vi "test Add RAF Channel.vi"(8 "error in (no error)":errorcluster, 11 "TestCase in":refnum<class "Switch Scripting Unit Tests.lvclass">) -> (0 "error out":errorcluster, 3 "TestCase out":refnum<class "Switch Scripting Unit Tests.lvclass">)   [LabVIEW 2017, in "Switch Scripting.lvlib" / "Switch Scripting Unit Tests.lvclass"]
uses:
  Switch Scripting Unit Tests.lvclass
  Channel States.ctl
  Routing State.ctl
  Routing Channel/Connection.ctl
  Switch Scripting Unit Tests.lvclass/Switch Scripting Unit Tests.ctl
  <vilib>/addons/_JKI Toolkits/VI Tester/TestCase.llb/TestCase.lvclass
  Switch Scripting.lvlib
  C:/Program Files (x86)/National Instruments/LabVIEW 2017/vi.lib/addons/_JKI Toolkits/VI Tester/TestCase.llb/TestCase.lvclass
panel:
  in  "Save?":bool
  out "Output Filename":string
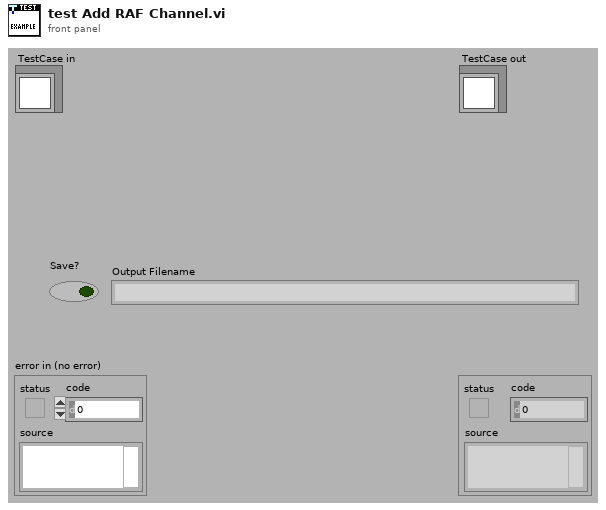
[diagram p1: front panel]
types:
  T1 = typedef "Switch Scripting.lvlib/Connection.ctl" = cluster{"source":string, "destination":string}
  T2 = typedef "Switch Scripting.lvlib/Channel States.ctl" = T3[]
  T3 = typedef "Switch Scripting.lvlib/Routing State.ctl" = cluster{"name":string, "description":string, "value":i32, "connection list":T1[]}
  T4 = typedef "Custom Device API.lvlib/Custom Device Item Ref.ctl" = u64
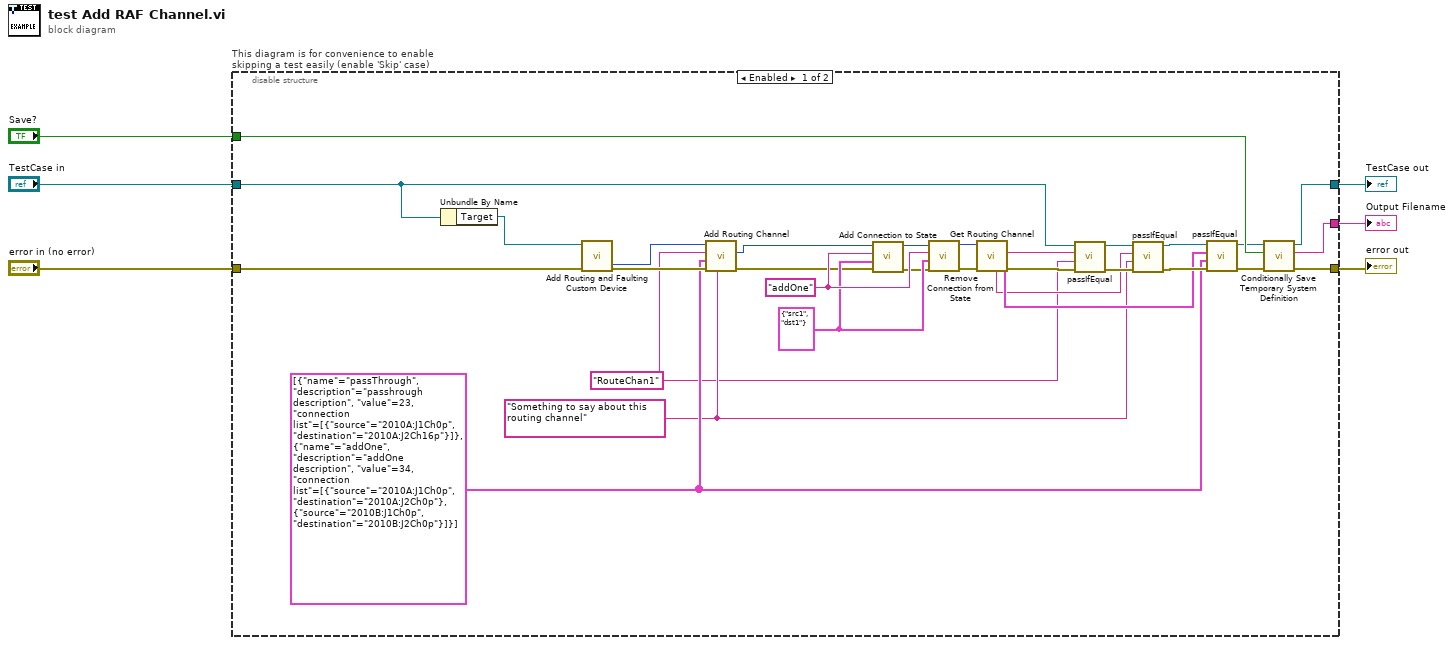
[diagram p0: block diagram]
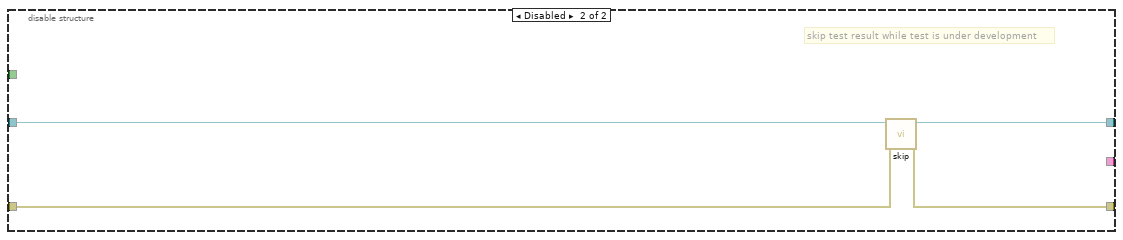
[diagram p2: hidden frame]
diagram:
  n1 = disable-structure "This diagram is for convenience to enable skipping a test easily (enable 'Skip' case)" shown="Enabled" {
    disable-tunnel: "TestCase in" -> [w16 w40]
    disable-tunnel: [w31 w38] -> w3
    disable-tunnel: [w35 w39] -> w5
    disable-tunnel: "error in (no error)" -> [w36 w37]
    disable-tunnel: [w34 _] -> w2
    disable-tunnel: "Save?" -> [w33 _]
    frame Enabled {
      w9 = "Something to say about this routing channel" ("Description")
      w25 = T1 {"source"="src1", "destination"="dst1"} ("connection")
      w26 = "addOne" ("state name")
      w11 = T2 [{"name"="passThrough", "description"="passhrough description", "value"=23, "connection list"=[{"source"="2010A:J1Ch0p", "destination"="2010A:J2Ch16p"}]}, {"name"="addOne", "description"="addOne description", "value"=34, "connection list"=[{"source"="2010A:J1Ch0p", "destination"="2010A:J2Ch0p"}, {"source"="2010B:J1Ch0p", "destination"="2010B:J2Ch0p"}]}] ("Channel States")
      w8 = "RouteChan1" ("Channel Name")
      n2 = Unbundle By Name(w16) -> ("Target"=w32:refnum<k24>)
      n3 = call "Add Routing and Faulting Custom Device.vi"("error in (no error)"=w36, "Target in"=w32) -> ("error out"=w30:errorcluster, "Routes Section Ref"=w21:T4)  [unwired: 5 in, 3 out]
      n4 = call "Add Routing Channel.vi"("Description"=w9, "error in (no error)"=w30, "States and Connections"=w11, "Channel Name"=w8, "Routes Ref in"=w21) -> ("error out"=w22:errorcluster, "Channel Ref"=w19:T4)  [unwired: 4 in, 1 out]
      n5 = call "Add Connection to State.vi"("error in (no error)"=w22, "Connection"=w25, "State"=w26, "Channel Ref in"=w19) -> ("error out"=w23:errorcluster, "Channel Ref out"=w27:T4)  [unwired: 6 in]
      n6 = call "Remove Connection from State.vi"("error in (no error)"=w23, "Connection"=w25, "State"=w26, "Channel Ref in"=w27) -> ("error out"=w24:errorcluster, "Channel Ref out"=w20:T4)  [unwired: 5 in, 1 out]
      n7 = call "Get Routing Channel.vi"("error in (no error)"=w24, "Channel Ref in"=w20) -> ("error out"=w14:errorcluster, "Channel States"=w12:T2, "Channel Name"=w7:string, "Description"=w10:string)  [unwired: 5 in, 1 out]
      n8 = call-dynamic "passIfEqual.vi"("error in (no error)"=w14, "y"=w8, "x"=w7, "TestCase in"=w16) -> ("error out"=w18:errorcluster, "TestCase out"=w17:refnum<class "Switch Scripting Unit Tests.lvclass">)  [unwired: 6 in]
      n9 = call-dynamic "passIfEqual.vi"("error in (no error)"=w18, "y"=w9, "x"=w10, "TestCase in"=w17) -> ("error out"=w13:errorcluster, "TestCase out"=w15:refnum<class "Switch Scripting Unit Tests.lvclass">)  [unwired: 6 in]
      n10 = call-dynamic "passIfEqual.vi"("error in (no error)"=w13, "y"=w11, "x"=w12, "TestCase in"=w15) -> ("error out"=w29:errorcluster, "TestCase out"=w28:refnum<class "Switch Scripting Unit Tests.lvclass">)  [unwired: 6 in]
      n11 = call "Conditionally Save Temporary System Definition.vi"("error in (no error)"=w29, "Save?"=w33, "Test Case"=w28) -> ("error out"=w35:errorcluster, "filename"=w34:string, "Test Case"=w31:refnum<class "Switch Scripting Unit Tests.lvclass">)  [unwired: 6 in]
    }
    frame Disabled {
      # "skip test result while test is under development"
      n12 = call <vilib>:"skip.vi"("error in (no error)"=w37, "TestCase in"=w40) -> ("error out"=w39:errorcluster, "TestCase out"=w38:refnum<class "Switch Scripting Unit Tests.lvclass">)  [unwired: 8 in]
    }
  }
  "error out" <- w5
  "TestCase out" <- w3
  "Output Filename" <- w2
